vi "Create All Message Queues.vi"(8 "error in (no error)":errorcluster) -> (0 "error out":errorcluster, 3 "Message Queues out":T1)   [LabVIEW 2020, in "Message Queue.lvlib"]
doc: "This VI creates and initializes all the message queues for your application. If your application requires more than one message queue, right-click the \"Message Queues\" constant above and select Open Type Def. Add the new Message Queue(s) to the type definition, then initialize them in this VI."
uses:
  Message Queue.lvlib
  All Message Queues.ctl
  Message Cluster.ctl
  Enqueue Message (Single).vi
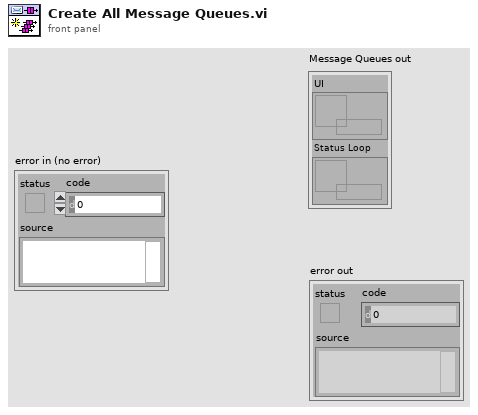
[diagram p1: front panel]
types:
  T1 = typedef "Message Queue.lvlib/All Message Queues.ctl" = cluster{"UI":refnum<queue>, "Status Loop":refnum<queue>}
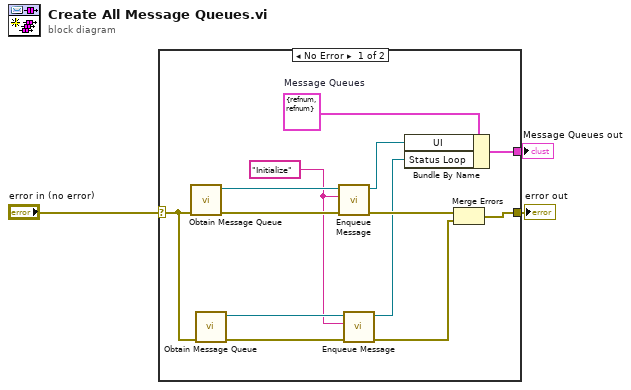
[diagram p0: block diagram]
diagram:
  n1 = case shown="No Error" "error in (no error)" {
    selector: "error in (no error)" -> [w10 w17]
    tunnel: [w6 w17] -> w3
    tunnel: [w15 _] -> w2
    frame No Error {
      w9 = "Initialize" ("Message")
      w16 = T1 {"UI"=refnum, "Status Loop"=refnum}  # Message Queues
      n2 = call "Obtain Message Queue.vi"("error in (no error)"=w10) -> ("error out"=w14:errorcluster, "Message Queue"=w13:refnum<queue>)  [unwired: 9 in]
      n3 = call "Obtain Message Queue.vi"("error in (no error)"=w10) -> ("error out"=w12:errorcluster, "Message Queue"=w11:refnum<queue>)  [unwired: 9 in]
      n4 = call-poly "Enqueue Message.vi"("error in (no error)"=w14, "Message"=w9, "Message Queue"=w13) -> ("error out"=w8:errorcluster, "dup Message Queue"=w4:refnum<queue>)  [unwired: 7 in]
      n5 = call-poly "Enqueue Message.vi"("error in (no error)"=w12, "Message"=w9, "Message Queue"=w11) -> ("error out"=w7:errorcluster, "dup Message Queue"=w5:refnum<queue>)  [unwired: 7 in]
      n6 = Bundle By Name(cluster=w16, "UI"=w4, "Status Loop"=w5) -> (w15:T1)
      n7 = Merge Errors(w8, w7) -> (w6:errorcluster)
    }
    frame Error {
    }
  }
  "Message Queues out" <- w2
  "error out" <- w3
